vi "Insight OCT.vi"() -> ()   [LabVIEW 2014]
doc: "I. Description:\nThis example demonstrates how to acquire a continuous amount of data (Waveform) using the DAQ device's internal clock.\n\nII. Instructions for Running:\n1. Create an analog input voltage channel.\n2. Set the rate for the sample clock. Additionally, define the sample mode to be continuous.\n3. Call the Start VI to start the acquisition.\n4. Read the waveform data in a loop until the user hits the stop button or an error occurs.\nNote: This example reads data from one or more channels and returns an array of data. Use the Index Array function to access an individual channel of data.\n5. Call the Clear Task VI to clear the Task.\n6. Use the popup dialog box to display an error if any.\n\nIV. I/O Connections Overview:\nMake sure your signal input terminal matches the Physical Channel I/O Control. For further connection information, refer to your hardware reference manual."
uses:
  Type Defs/OCT Hardware States.ctl
  Classes/DAQ/DAQ Control Functional Global States.ctl
  Classes/Processing/Intensity/Intensity Processing.lvclass
  Classes/Galvo/NI Galvo/NI Galvo.lvclass
  Classes/DAQ/DAQ Class.lvclass
  Classes/DAQ/ATS9350/ATS9350.lvclass
  Classes/Laser/Insite/Insight.lvclass
  Type Defs/OCT DAQ Channel Data Type.ctl
  Classes/Galvo/Scanning Cluster.ctl
  Classes/Galvo/Galvo.lvclass
  Classes/DAQ/Clock Control.ctl
  Classes/DAQ/Trigger Source.ctl
  Classes/DAQ/Trigger Slope.ctl
  Classes/DAQ/DAQ Parameters.ctl
panel:
  out "Initial DAQ Parameters":T1={"Points Per A-Scan"=1024, "A-Scans Per B-Scan"=250, "Number of B-Scans"=1, "A-Scans Per Transfer"=1, "Trigger Voltage"=0.0, "Trigger Source"=enum."External", "Trigger Slope"=enum."Rising", "Channel"=enum."Channel 1", "Clock"=enum."Internal Clock", "Bits per Sample"=0.0, "Range"=0.0}
  in  "Laser Status":string
  out "Single A-Scan":u16[](graph)
  in  "Scanning Parameters":T6={"Fast Axis Offset"=0.0, "Slow Axis Offset"=0.0, "Slow Axis Amp"=2.0, "Fast Axis Amp"=2.0, "Scan Pattern"=enum."Raster"} {"Fast Axis Amp" max=20 format="%#.2f"; "Slow Axis Amp" max=20 format="%#.2f"; "Slow Axis Offset" max=10 format="%#.2f"; "Fast Axis Offset" max=10 format="%#.2f"}
  out "Log10?":bool
  in  "OCT Hardware States":T7
  out "Background Array":u16[](array[numeric])
  in  "Save Sweep Button":bool
  in  "Data Format":T4
  in  "Save Sweep":bool
  in  "Stop Button":bool
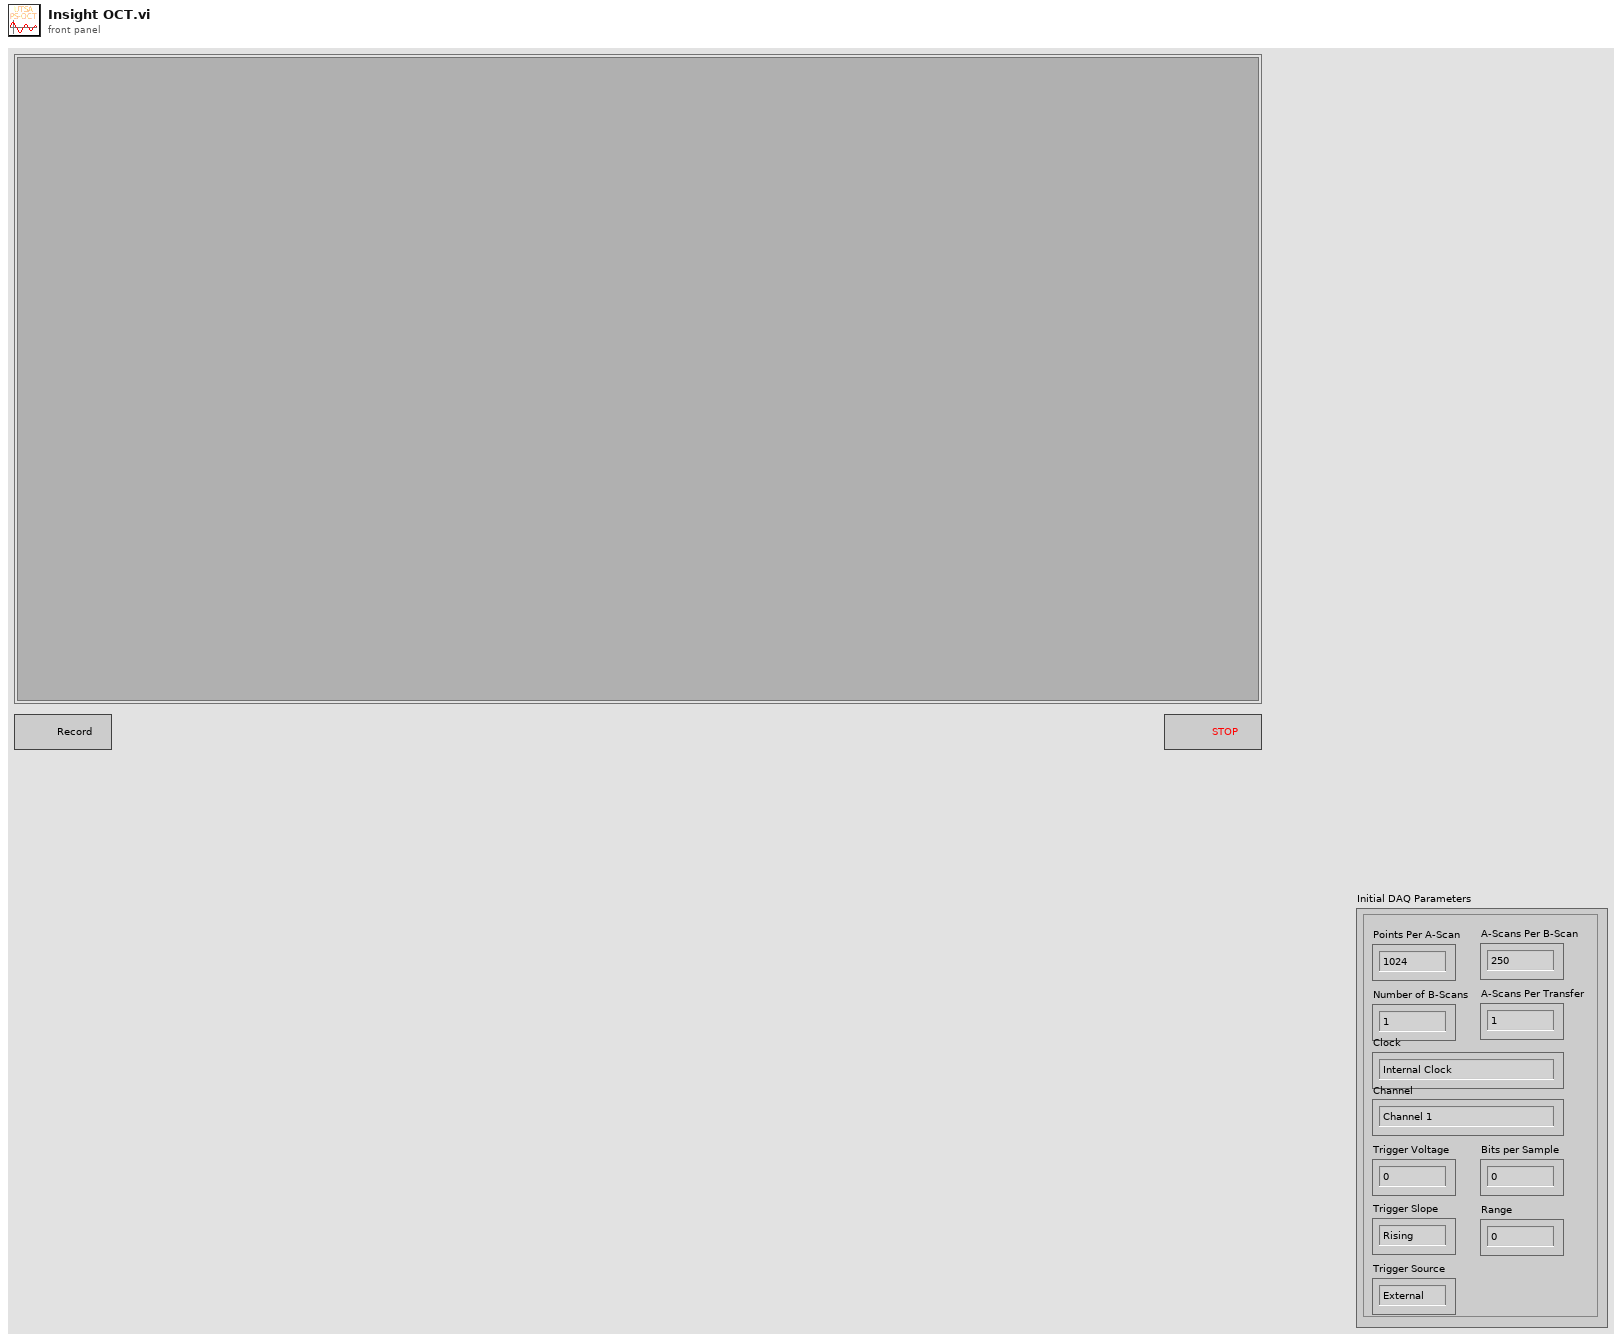
[diagram p1: front panel]
types:
  T1 = typedef "DAQ Class.lvclass/DAQ Parameters.ctl" = cluster{"Points Per A-Scan":u32, "A-Scans Per B-Scan":u32, "Number of B-Scans":u32, "A-Scans Per Transfer":u32, "Trigger Voltage":sgl, "Trigger Source":T2, "Trigger Slope":T3, "Channel":T4, "Clock":T5, "Bits per Sample":dbl, "Range":dbl}
  T2 = typedef "DAQ Class.lvclass/Trigger Source.ctl" = enum16{"External", "Channel A", "Channel B"}
  T3 = typedef "DAQ Class.lvclass/Trigger Slope.ctl" = enum16{"Rising", "Falling"}
  T4 = typedef "OCT DAQ Channel Data Type.ctl" = enum16{"Channel 1", "Channel 2", "Channel 1 and 2"}
  T5 = typedef "DAQ Class.lvclass/Clock Control.ctl" = enum16{"Internal Clock", "External Clock"}
  T6 = typedef "Galvo.lvclass/Scanning Cluster.ctl" = cluster{"Fast Axis Offset":sgl, "Slow Axis Offset":sgl, "Slow Axis Amp":sgl, "Fast Axis Amp":sgl, "Scan Pattern":enum16{"Raster"}}
  T7 = typedef "OCT Hardware States.ctl" = enum16{"Acquire Data", "Initialize Laser", "Initialize Galvos", "Startup", "Reset DAQ", "Background Subtraction", "Acquire Background", "Update DAQ Parameters", "Stop", "Set Clock", "Initialize DAQ", "Set Resampling Array", "Save Sweep", "Configure Laser", "128 x 128", "512 x 1", "512 x 512", "Review Data", "Configure Trigger", "Update Galvos"}
  T8 = typedef "DAQ Control Functional Global States.ctl" = enum16{"Status", "Set Processing Finished", "Reset", "Clear", "Set DAQ Finished"}
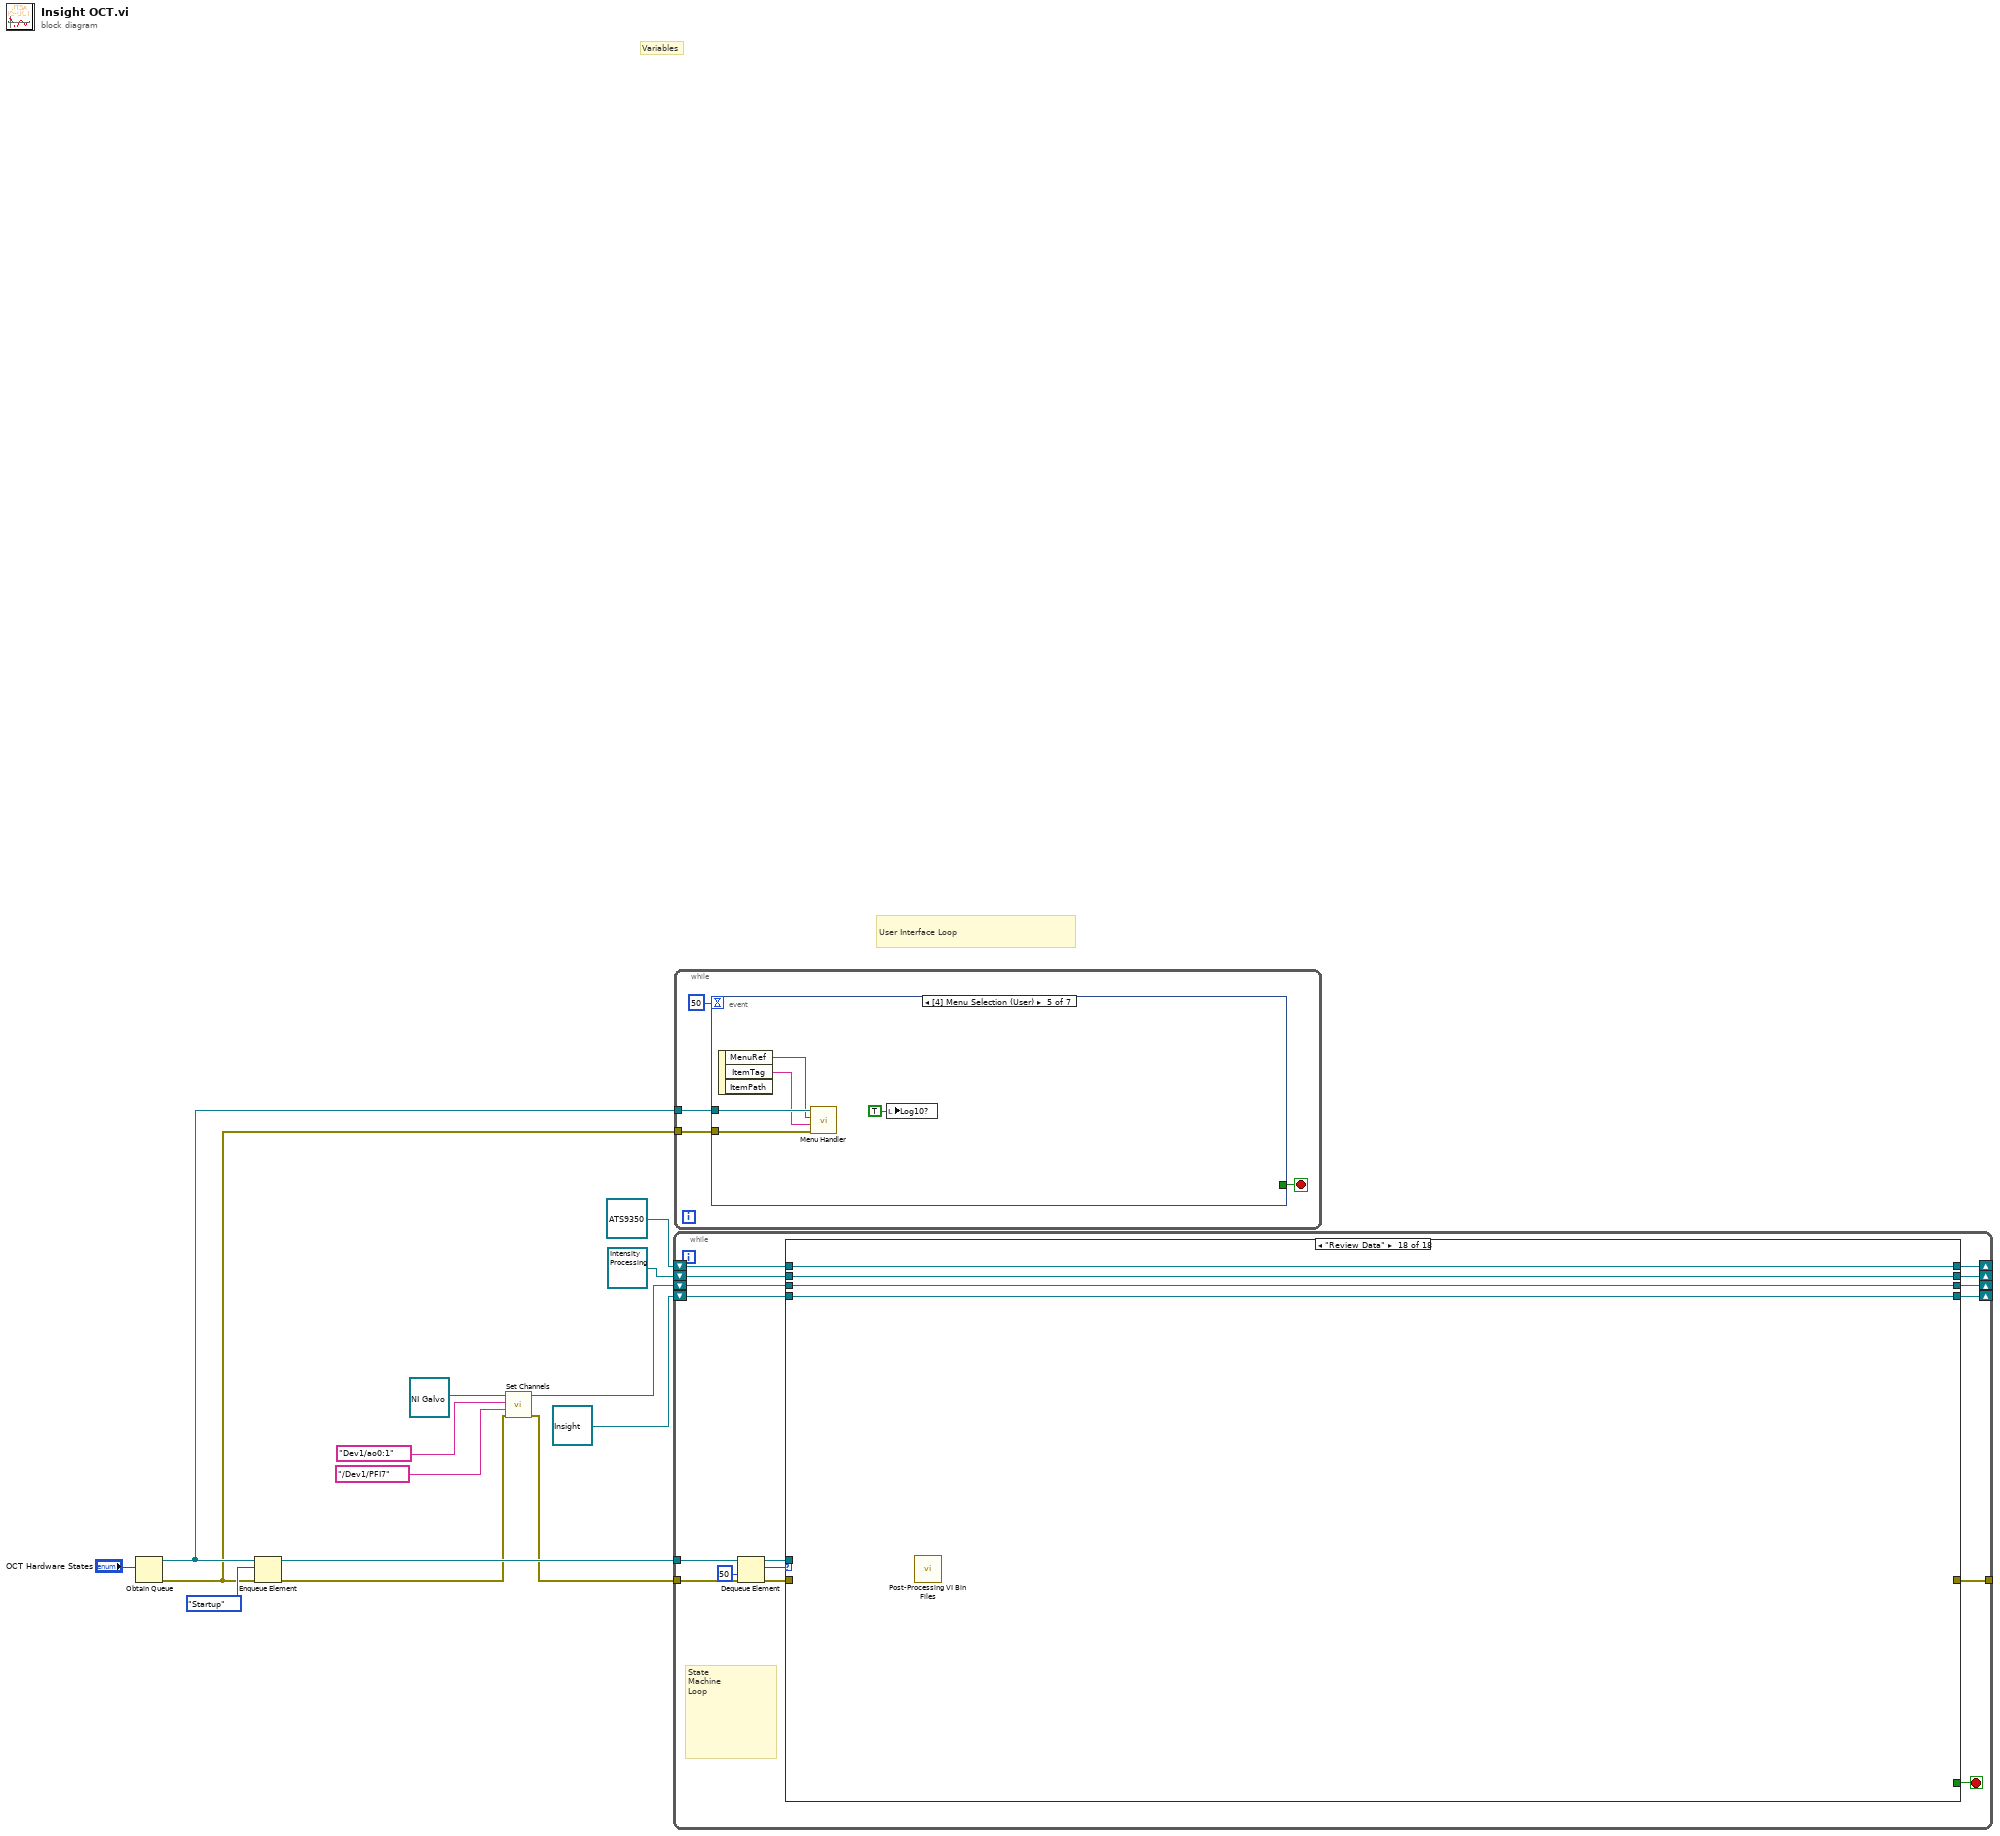
[diagram p0: block diagram]
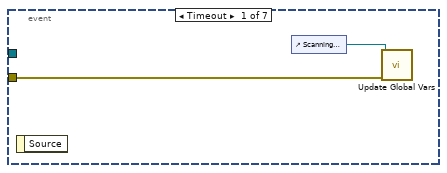
[diagram p2: hidden frame]
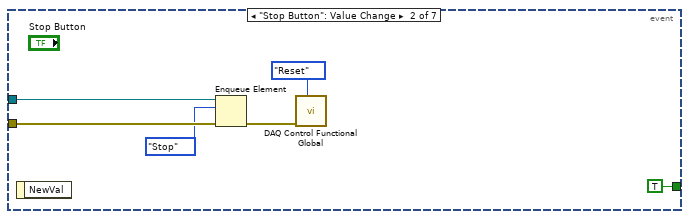
[diagram p3: hidden frame]
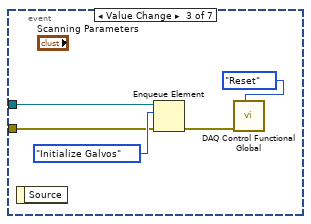
[diagram p4: hidden frame]
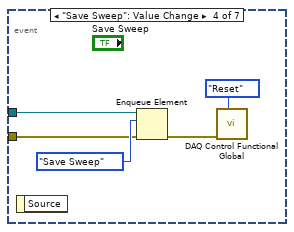
[diagram p5: hidden frame]
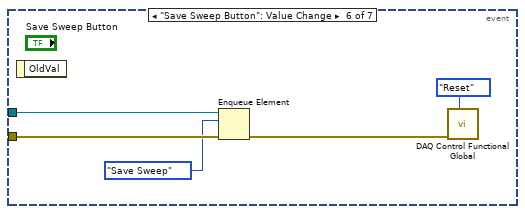
[diagram p6: hidden frame]
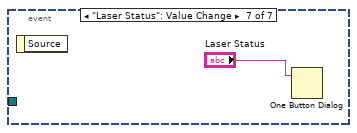
[diagram p7: hidden frame]
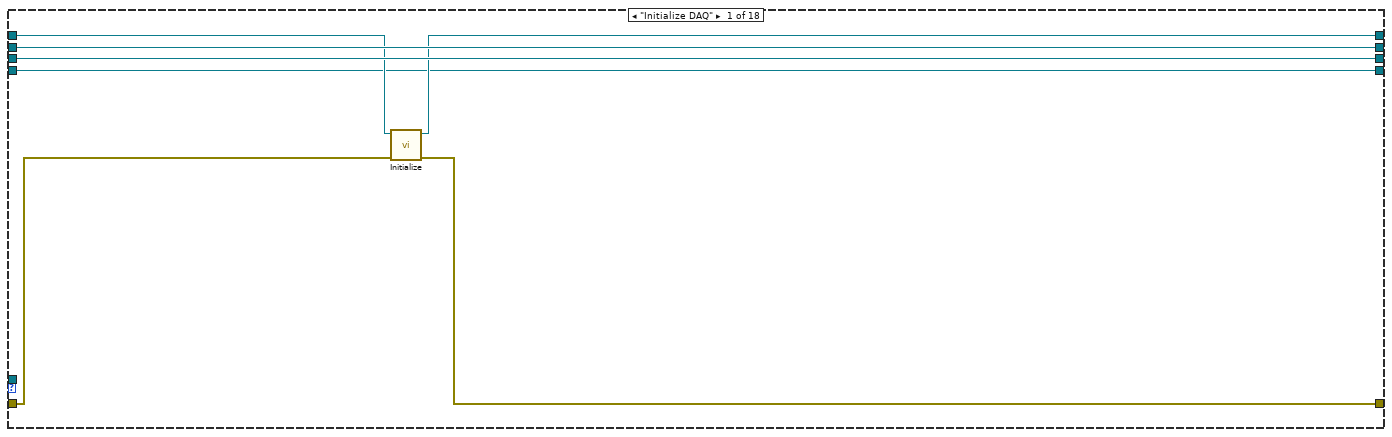
[diagram p8: hidden frame]
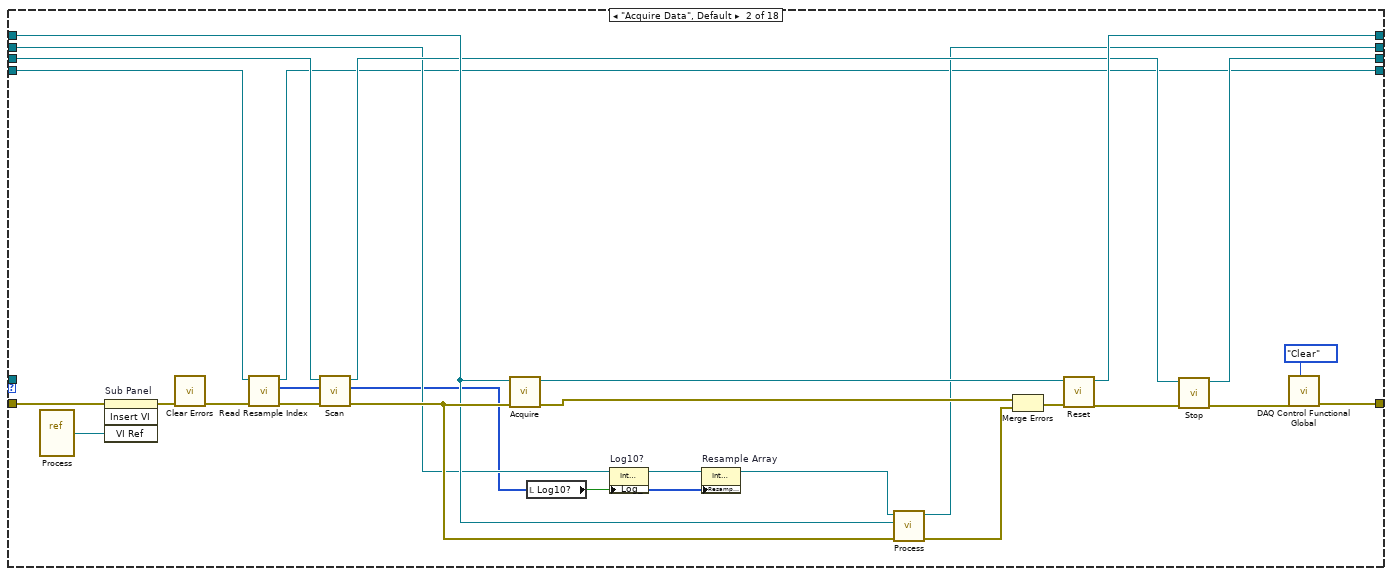
[diagram p9: hidden frame]
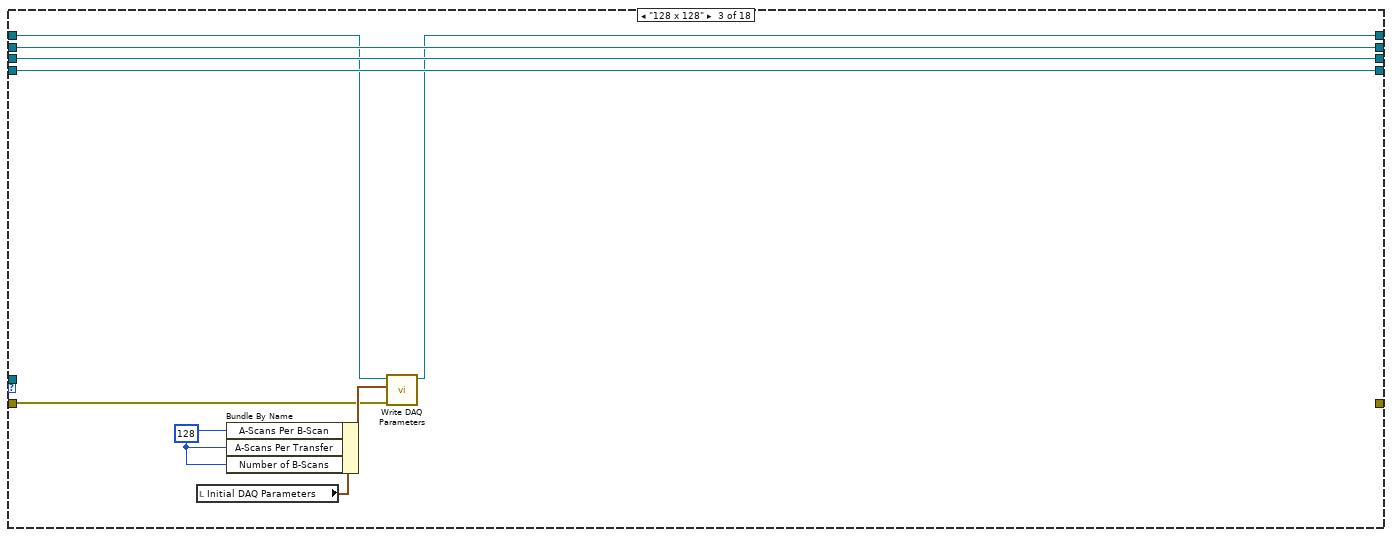
[diagram p10: hidden frame]
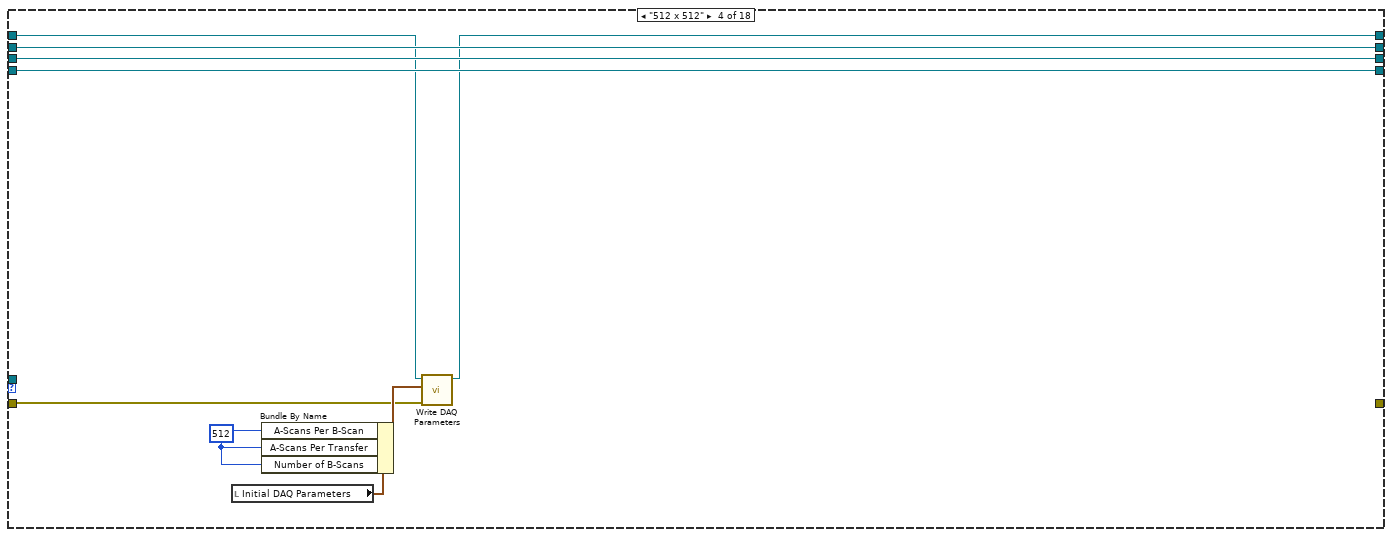
[diagram p11: hidden frame]
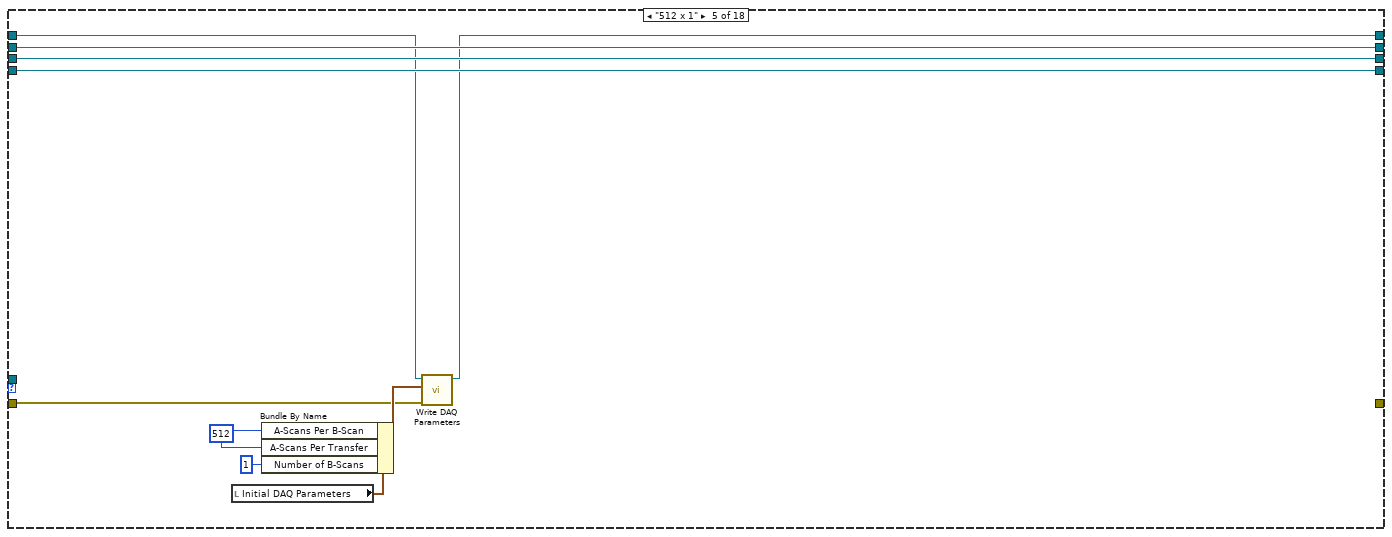
[diagram p12: hidden frame]
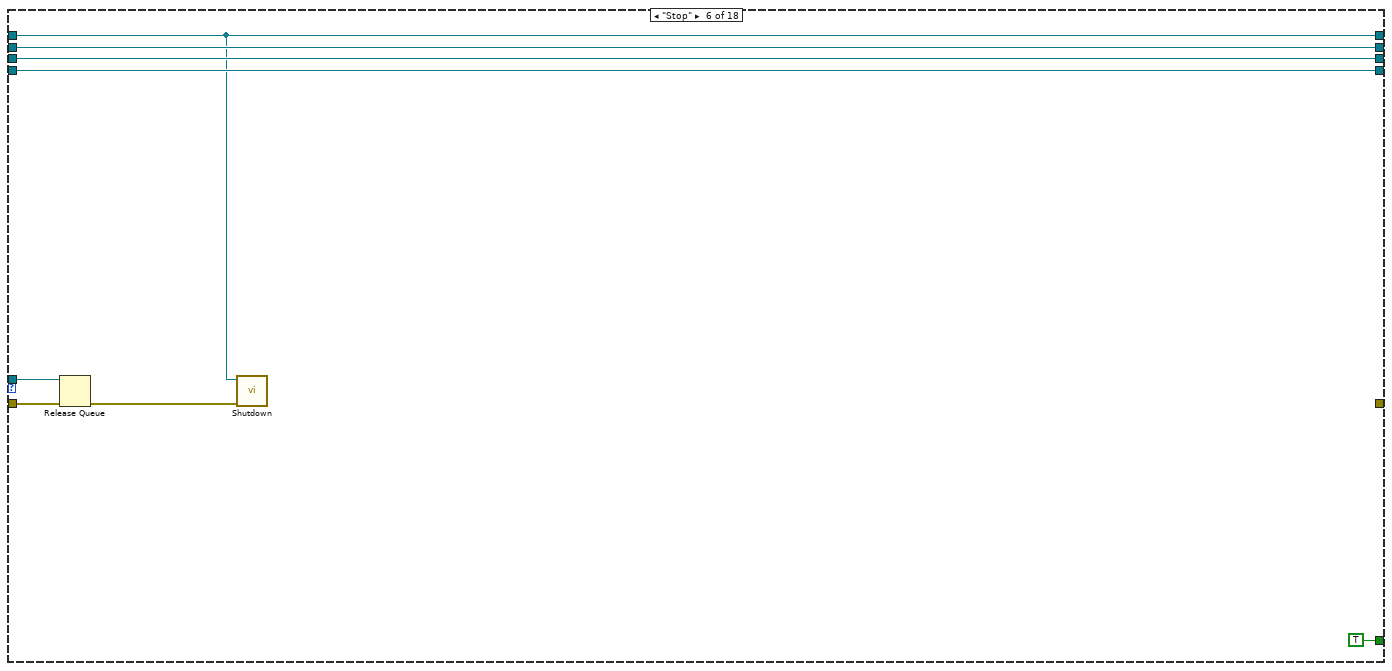
[diagram p13: hidden frame]
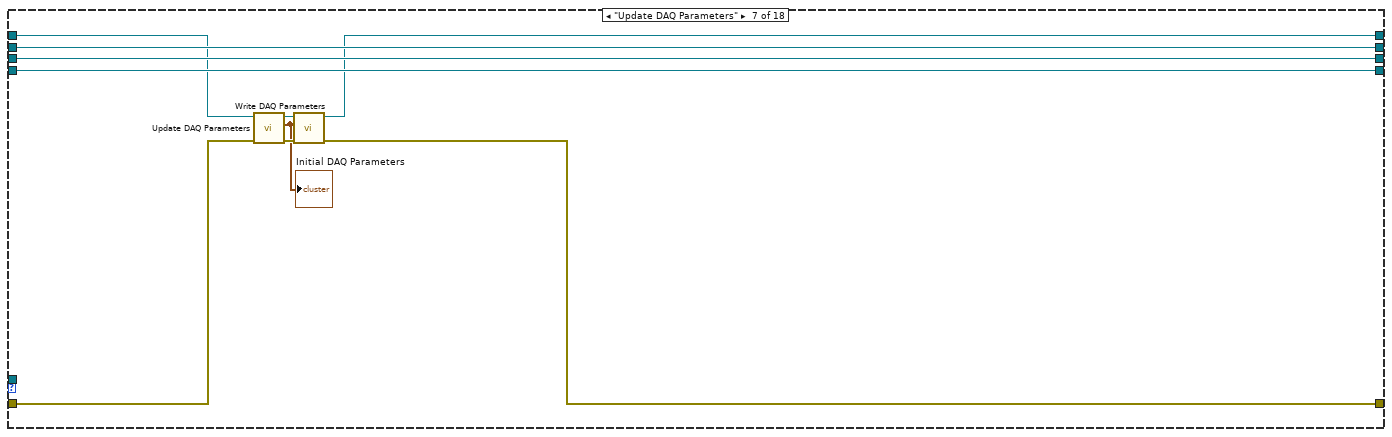
[diagram p14: hidden frame]
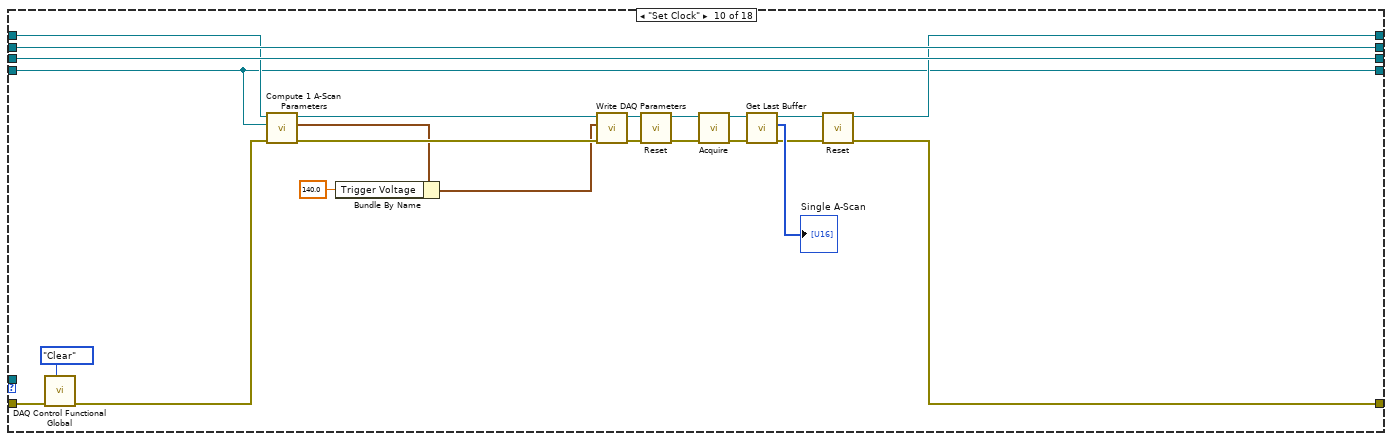
[diagram p17: hidden frame]
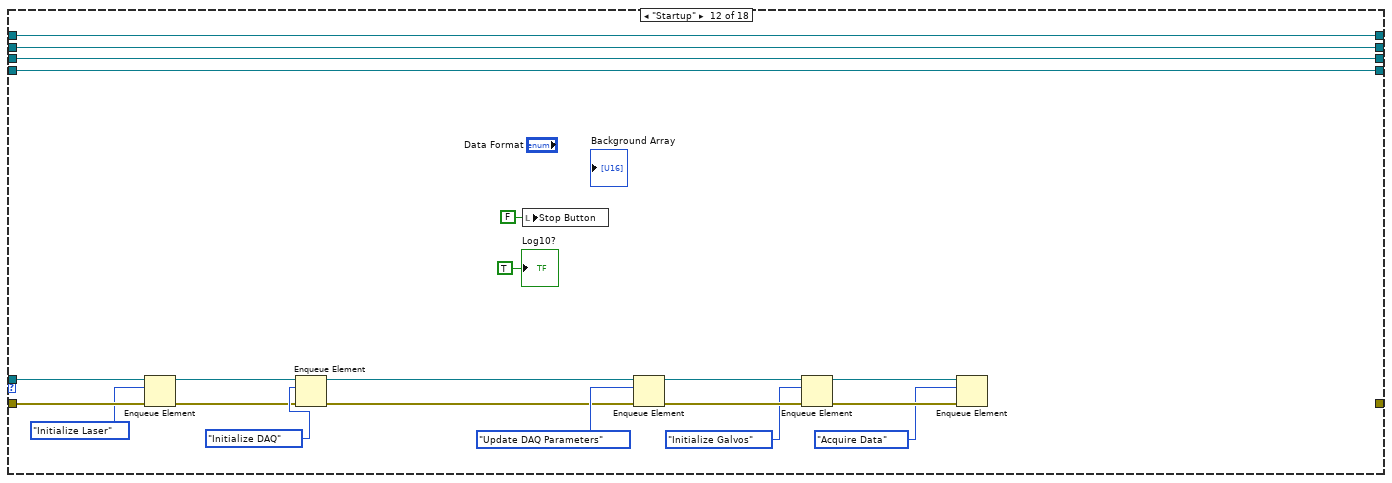
[diagram p19: hidden frame]
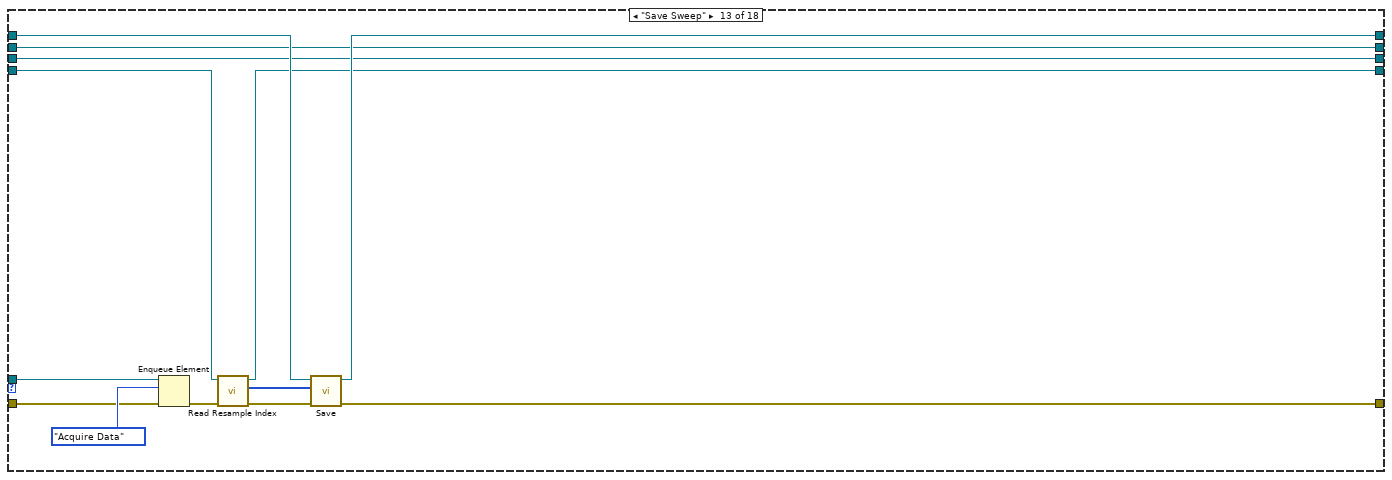
[diagram p20: hidden frame]
diagram:
  # "User Interface Loop"
  # "Variables"
  n1 = Obtain Queue(element data type="OCT Hardware States") -> (queue out=w12:refnum<queue>, error out=w10:errorcluster)  [unwired: 4 in, 1 out]
  n2 = Enqueue Element(queue=w12, element=OCT_Hardware_States."Startup", error in (no error)=w10) -> (queue out=w13:refnum<queue>, error out=w7:errorcluster)  [unwired: 1 in, 1 out]
  n3 = call-dynamic "Set Channels.vi"("error in (no error)"=w7, "Trigger Source"=tag "/Dev1/PFI7", "Analog Output"=tag "Dev1/ao0:1", "NI Galvo in"=refnum<class "NI Galvo.lvclass"> refnum ("NI Galvo.lvclass")) -> ("error out"=w6:errorcluster, "NI Galvo out"=w5:refnum<class "NI Galvo.lvclass">)  [unwired: 6 in]
  n4 = while {
    tunnel: w13 -> [w30]
    tunnel: w6 -> [w25]
    tunnel: [w26] -> _
    shift-right: [w22] -> _
    shift-left: refnum<class "ATS9350.lvclass"> refnum ("ATS9350.lvclass") -> [w23]
    shift-right: [w18] -> _
    shift-left: refnum<class "Intensity Processing.lvclass"> refnum ("Intensity Processing.lvclass") -> [w21]
    shift-right: [w17] -> _
    shift-left: w5 -> [w20]
    shift-right: [w16] -> _
    shift-left: refnum<class "Insight.lvclass"> refnum ("Insight.lvclass") -> [w19]
    stop <- w15 stop-if-true
    # "State\nMachine\nLoop"
    n5 = Dequeue Element(queue=w30, timeout in ms (-1)=50, error in (no error)=w25) -> (queue out=w28:refnum<queue>, element=w24:T7, error out=w29:errorcluster)  [unwired: 1 out]
    n6 = case shown="\"Review Data\"" w24 {
      tunnel: w29 -> [w32 w54 w67 w76 w86 w99 w110 _ _ w138 _ w151 w178 w186 _ w200 w210 _]
      tunnel: w28 -> [_ _ _ _ _ w100 _ _ _ _ _ w152 w177 _ _ _ _ _]
      tunnel: [w37 w63 _ _ _ _ w102 _ _ w120 _ _ w176 w189 _ w198 w205 _] -> w26
      tunnel: w23 -> [w34 w51 w66 w75 w85 w94 w104 w114 w118 w128 w145 w156 w175 w181 w196 w203 w213 w217]
      tunnel: [w33 w50 w65 w74 w84 w94 w103 w114 w118 w121 w145 w156 w174 w180 w196 w203 w213 w217] -> w22
      tunnel: w21 -> [w36 w47 w73 w82 w92 w97 w107 w113 w117 w130 w144 w155 w173 w185 w195 w202 w212 w216]
      tunnel: w20 -> [w35 w52 w72 w81 w91 w96 w106 w112 w116 w129 w143 w154 w172 w183 w194 w201 w211 w215]
      tunnel: w19 -> [w31 w42 w71 w80 w90 w95 w105 w111 w115 w119 w142 w153 w169 w184 w193 w199 w207 w214]
      tunnel: [w36 w46 w73 w82 w92 w97 w107 w113 w117 w130 w144 w155 w173 w185 w195 w202 w212 w216] -> w18
      tunnel: [w35 w48 w72 w81 w91 w96 w106 w112 w116 w129 w143 w154 w172 w182 w194 w201 w211 w215] -> w17
      tunnel: [w31 w41 w71 w80 w90 w95 w105 w111 w115 w119 w142 w153 w168 w184 w193 w197 w206 w214] -> w16
      tunnel: [_ _ _ _ _ TRUE _ _ _ _ _ _ _ _ _ _ _ _] -> w15
      frame "Initialize DAQ" {
        n7 = call-dynamic "Initialize.vi"("error in (no error)"=w32, "ATS9350 in"=w34) -> ("error out"=w37:errorcluster, "ATS9350 out"=w33:refnum<class "ATS9350.lvclass">)  [unwired: 8 in]
      }
      frame "Acquire Data", Default {
        n8 = vi-ref "Process.vi"() -> (w53:refnum<vi>)
        n9 = invoke on="Sub Panel" class="SubPanel" method="Insert VI"(error in=w54, "VI Ref"=w53) -> (error out=w45:errorcluster)  [unwired: 2 in, 3 out]
        n10 = call <vilib>:"Clear Errors.vi"("error in (no error)"=w45) -> ("error out"=w44:errorcluster)  [unwired: 5 in, 1 out]
        n11 = call-dynamic "Read Resample Index.vi"("error in (no error)"=w44, "Laser in"=w42) -> ("error out"=w43:errorcluster, "Resample Index"=w39:u32[], "Laser out"=w41:refnum<class "Insight.lvclass">)  [unwired: 7 in]
        n12 = call-dynamic "Scan.vi"("error in (no error)"=w43, "NI Galvo in"=w52) -> ("error out"=w57:errorcluster, "NI Galvo out"=w49:refnum<class "NI Galvo.lvclass">)  [unwired: 8 in]
        n13 = call-dynamic "Acquire.vi"("error in (no error)"=w57, "ATS9350 in"=w51) -> ("error out"=w61:errorcluster, "ATS9350 out"=w59:refnum<class "ATS9350.lvclass">)  [unwired: 8 in]
        n14 = local read "Log10?"() -> (w58:bool)
        n15 = property on="Log10?" class="Intensity Processing.lvclass"(reference=w47, "Log_"=w58) -> (reference out=w40:refnum<class "Intensity Processing.lvclass">)  [unwired: 1 in, 1 out]
        n16 = property on="Resample Array" class="Intensity Processing.lvclass"(reference=w40, "Resample Array"=w39) -> (reference out=w38:refnum<class "Intensity Processing.lvclass">)  [unwired: 1 in, 1 out]
        n17 = call-dynamic "Process.vi"("error in (no error)"=w57, "DAQ Class.lvclass"=w51, "Intensity Processing in"=w38) -> ("error out"=w62:errorcluster, "Intensity Processing out"=w46:refnum<class "Intensity Processing.lvclass">)  [unwired: 7 in]
        n18 = Merge Errors(w61, w62) -> (w60:errorcluster)
        n19 = call-dynamic "Reset.vi"("error in (no error)"=w60, "ATS9350 in"=w59) -> ("error out"=w56:errorcluster, "ATS9350 out"=w50:refnum<class "ATS9350.lvclass">)  [unwired: 8 in]
        n20 = call-dynamic "Stop.vi"("error in (no error)"=w56, "NI Galvo in"=w49) -> ("error out"=w55:errorcluster, "NI Galvo out"=w48:refnum<class "NI Galvo.lvclass">)  [unwired: 8 in]
        n21 = call "DAQ Control Functional Global.vi"("State"=DAQ_Control_Functional_Global_States."Clear", "Error In"=w55) -> ("Error Out"=w63:errorcluster)  [unwired: 6 in, 3 out]
      }
      frame "128 x 128" {
        w69 = u32 128 ("A-Scans Per B-Scan")
        n22 = local read "Initial DAQ Parameters"() -> (w70:T1)
        n23 = Bundle By Name(cluster=w70, "A-Scans Per B-Scan"=w69, "A-Scans Per Transfer"=w69, "Number of B-Scans"=w69) -> (w68:T1)
        n24 = call-dynamic "Write DAQ Parameters.vi"("error in (no error)"=w67, "DAQ Parameters"=w68, "ATS9350 in"=w66) -> ("ATS9350 out"=w65:refnum<class "ATS9350.lvclass">)  [unwired: 7 in, 1 out]
      }
      frame "512 x 512" {
        w78 = u32 512 ("A-Scans Per B-Scan")
        n25 = local read "Initial DAQ Parameters"() -> (w79:T1)
        n26 = Bundle By Name(cluster=w79, "A-Scans Per B-Scan"=w78, "A-Scans Per Transfer"=w78, "Number of B-Scans"=w78) -> (w77:T1)
        n27 = call-dynamic "Write DAQ Parameters.vi"("error in (no error)"=w76, "DAQ Parameters"=w77, "ATS9350 in"=w75) -> ("ATS9350 out"=w74:refnum<class "ATS9350.lvclass">)  [unwired: 7 in, 1 out]
      }
      frame "512 x 1" {
        w88 = u32 512 ("A-Scans Per B-Scan")
        n28 = local read "Initial DAQ Parameters"() -> (w89:T1)
        n29 = Bundle By Name(cluster=w89, "A-Scans Per B-Scan"=w88, "A-Scans Per Transfer"=w88, "Number of B-Scans"=u32 1) -> (w87:T1)
        n30 = call-dynamic "Write DAQ Parameters.vi"("error in (no error)"=w86, "DAQ Parameters"=w87, "ATS9350 in"=w85) -> ("ATS9350 out"=w84:refnum<class "ATS9350.lvclass">)  [unwired: 7 in, 1 out]
      }
      frame "Stop" {
        n31 = Release Queue(queue=w100, error in (no error)=w99) -> (error out=w98:errorcluster)  [unwired: 1 in, 2 out]
        n32 = call-dynamic "Shutdown.vi"("error in (no error)"=w98, "ATS9350 in"=w94) -> ()  [unwired: 8 in, 2 out]
      }
      frame "Update DAQ Parameters" {
        n33 = call-dynamic "Update DAQ Parameters.vi"("error in (no error)"=w110, "DAQ Class in"=w104) -> ("error out"=w108:errorcluster, "DAQ Parameters Out"=w101:T1, "DAQ Class out"=w109:refnum<class "ATS9350.lvclass">)  [unwired: 7 in]
        "Initial DAQ Parameters" <- w101
        n34 = call-dynamic "Write DAQ Parameters.vi"("error in (no error)"=w108, "DAQ Parameters"=w101, "ATS9350 in"=w109) -> ("error out"=w102:errorcluster, "ATS9350 out"=w103:refnum<class "ATS9350.lvclass">)  [unwired: 7 in]
      }
      frame "Background Subtraction" {
      }
      frame "Acquire Background" {
      }
      frame "Set Clock" {
        n35 = call "DAQ Control Functional Global.vi"("State"=DAQ_Control_Functional_Global_States."Clear", "Error In"=w138) -> ("Error Out"=w137:errorcluster)  [unwired: 6 in, 3 out]
        n36 = call "Compute 1 A-Scan Parameters.vi"("error in (no error)"=w137, "Laser In"=w119, "DAQ Class.lvclass"=w128) -> ("error out"=w131:errorcluster, "DAQ Parameters"=w127:T1, "DAQ Class.lvclass 2"=w132:refnum<class "ATS9350.lvclass">)  [unwired: 6 in]
        n37 = Bundle By Name(cluster=w127, "Trigger Voltage"=sgl 140.0) -> (w125:T1)
        n38 = call-dynamic "Write DAQ Parameters.vi"("error in (no error)"=w131, "DAQ Parameters"=w125, "ATS9350 in"=w132) -> ("error out"=w136:errorcluster, "ATS9350 out"=w135:refnum<class "ATS9350.lvclass">)  [unwired: 7 in]
        n39 = call-dynamic "Reset.vi"("error in (no error)"=w136, "ATS9350 in"=w135) -> ("error out"=w133:errorcluster, "ATS9350 out"=w134:refnum<class "ATS9350.lvclass">)  [unwired: 8 in]
        n40 = call-dynamic "Acquire.vi"("error in (no error)"=w133, "ATS9350 in"=w134) -> ("error out"=w140:errorcluster, "ATS9350 out"=w141:refnum<class "ATS9350.lvclass">)  [unwired: 8 in]
        n41 = call-dynamic "Get Last Buffer.vi"("error in (no error)"=w140, "DAQ Class in"=w141) -> ("error out"=w123:errorcluster, "Last Buffer"=→"Single A-Scan":u16[], "DAQ Class out"=w122:refnum<class "ATS9350.lvclass">)  [unwired: 7 in]
        n42 = call-dynamic "Reset.vi"("error in (no error)"=w123, "ATS9350 in"=w122) -> ("error out"=w120:errorcluster, "ATS9350 out"=w121:refnum<class "ATS9350.lvclass">)  [unwired: 8 in]
      }
      frame "Set Resampling Array" {
      }
      frame "Startup" {
        n43 = Enqueue Element(queue=w152, element=OCT_Hardware_States."Initialize Laser", error in (no error)=w151) -> (queue out=w149:refnum<queue>, error out=w150:errorcluster)  [unwired: 1 in, 1 out]
        n44 = Enqueue Element(queue=w149, element=OCT_Hardware_States."Initialize DAQ", error in (no error)=w150) -> (queue out=w147:refnum<queue>, error out=w146:errorcluster)  [unwired: 1 in, 1 out]
        n45 = local write "Stop Button"(FALSE ("Sweep Ready for saving")) -> ()
        n46 = Enqueue Element(queue=w147, element=OCT_Hardware_States."Update DAQ Parameters", error in (no error)=w146) -> (queue out=w164:refnum<queue>, error out=w163:errorcluster)  [unwired: 1 in, 1 out]
        n47 = Enqueue Element(queue=w164, element=OCT_Hardware_States."Initialize Galvos", error in (no error)=w163) -> (queue out=w159:refnum<queue>, error out=w158:errorcluster)  [unwired: 1 in, 1 out]
        n48 = Enqueue Element(queue=w159, element=OCT_Hardware_States."Acquire Data", error in (no error)=w158) -> ()  [unwired: 1 in, 3 out]
        "Log10?" <- TRUE ("Log10?")
      }
      frame "Save Sweep" {
        n49 = Enqueue Element(queue=w177, element=OCT_Hardware_States."Acquire Data", error in (no error)=w178) -> (error out=w171:errorcluster)  [unwired: 1 in, 2 out]
        n50 = call-dynamic "Read Resample Index.vi"("error in (no error)"=w171, "Laser in"=w169) -> ("error out"=w170:errorcluster, "Resample Index"=w167:u32[], "Laser out"=w168:refnum<class "Insight.lvclass">)  [unwired: 7 in]
        n51 = call-dynamic "Save.vi"("error in (no error)"=w170, "Resampling Array"=w167, "DAQ Class in"=w175) -> ("error out"=w176:errorcluster, "DAQ Class out"=w174:refnum<class "ATS9350.lvclass">)  [unwired: 7 in]
      }
      frame "Initialize Galvos" {
        n52 = call-dynamic "Read DAQ Parameters.vi"("error in (no error)"=w186, "ATS9350 in"=w181) -> ("error out"=w187:errorcluster, "DAQ Parameters"=w188:T1, "ATS9350 out"=w180:refnum<class "ATS9350.lvclass">)  [unwired: 7 in]
        n53 = local read "Scanning Parameters"() -> (w192:T6)
        n54 = call-dynamic "Configure.vi"("error in (no error)"=w187, "DAQ Parameters"=w188, "Scanning Parameters"=w192, "NI Galvo in"=w183) -> ("error out"=w191:errorcluster, "NI Galvo out"=w190:refnum<class "NI Galvo.lvclass">)  [unwired: 6 in]
        n55 = call-dynamic "Initialize.vi"("error in (no error)"=w191, "NI Galvo in"=w190) -> ("error out"=w189:errorcluster, "NI Galvo out"=w182:refnum<class "NI Galvo.lvclass">)  [unwired: 8 in]
      }
      frame "Reset DAQ" {
      }
      frame "Configure Laser" {
        n56 = call-dynamic "Configure.vi"("error in (no error)"=w200, "Insight in"=w199) -> ("error out"=w198:errorcluster, "Insight out"=w197:refnum<class "Insight.lvclass">)  [unwired: 8 in]
      }
      frame "Initialize Laser" {
        n57 = call-dynamic "Init.vi"("error in (no error)"=w210, "Insite in"=w207) -> ("error out"=w208:errorcluster, "Insite out"=w209:refnum<class "Insight.lvclass">)  [unwired: 8 in]
        n58 = call-dynamic "Read Status.vi"("error in (no error)"=w208, "Laser in"=w209) -> ("error out"=w205:errorcluster, "Status"=w204:string, "Laser out"=w206:refnum<class "Insight.lvclass">)  [unwired: 7 in]
        n59 = local write "Laser Status"(w204) -> ()
      }
      frame "Review Data" {
        n60 = call "Post-Processing VI Bin Files.vi"() -> ()  [unwired: 12 in]
      }
    }
  }
  n61 = while {
    tunnel: w12 -> [w221]
    tunnel: w10 -> [w220]
    stop <- w218 stop-if-true
    n62 = event shown="[4] Menu Selection (User)" {
      selector: _ -> [_ _ _ _ _ _ _]
      dyn-events: _ -> [_ _ _ _ _ _ _]
      timeout: 50 -> [_ _ _ _ _ _ _]
      tunnel: w221 -> [_ w228 w231 w236 w244 w246 _]
      tunnel: w220 -> [w222 w229 w232 w237 w243 w248 _]
      tunnel: [_ TRUE _ _ _ _ _] -> w218
      event Timeout {
        n63 = event-data() -> ()  [unwired: 1 in, 1 out]
        n64 = control-ref of="Scanning Parameters"() -> (w223:refnum<vi>)
        n65 = call "Update Global Vars.vi"("Error In"=w222, "Cluster in"=w223) -> ()  [unwired: 9 in, 1 out]
      }
      event "Stop Button": Value Change {
        n66 = event-data() -> ()  [unwired: 1 in, 1 out]
        n67 = Enqueue Element(queue=w228, element=OCT_Hardware_States."Stop", error in (no error)=w229) -> (error out=w226:errorcluster)  [unwired: 1 in, 2 out]
        n68 = call "DAQ Control Functional Global.vi"("State"=DAQ_Control_Functional_Global_States."Reset", "Error In"=w226) -> ()  [unwired: 6 in, 4 out]
      }
      event Value Change {
        n69 = event-data() -> ()  [unwired: 1 in, 1 out]
        n70 = Enqueue Element(queue=w231, element=OCT_Hardware_States."Initialize Galvos", error in (no error)=w232) -> (error out=w233:errorcluster)  [unwired: 1 in, 2 out]
        n71 = call "DAQ Control Functional Global.vi"("State"=DAQ_Control_Functional_Global_States."Reset", "Error In"=w233) -> ()  [unwired: 6 in, 4 out]
      }
      event "Save Sweep": Value Change {
        n72 = event-data() -> ()  [unwired: 1 in, 1 out]
        n73 = Enqueue Element(queue=w236, element=OCT_Hardware_States."Save Sweep", error in (no error)=w237) -> (error out=w235:errorcluster)  [unwired: 1 in, 2 out]
        n74 = call "DAQ Control Functional Global.vi"("State"=DAQ_Control_Functional_Global_States."Reset", "Error In"=w235) -> ()  [unwired: 6 in, 4 out]
      }
      event Menu Selection (User) {
        n75 = event-data() -> ("MenuRef"=w241:refnum<k9>, "ItemTag"=w242:string)  [unwired: 1 in, 1 out]
        n76 = call "Menu Handler.vi"("error in (no error)"=w243, "ItemTag"=w242, "Menu in"=w241, "queue in"=w244) -> ()  [unwired: 6 in, 2 out]
        n77 = local write "Log10?"(TRUE ("Log10?")) -> ()
      }
      event "Save Sweep Button": Value Change {
        n78 = event-data() -> ()  [unwired: 1 in, 1 out]
        n79 = Enqueue Element(queue=w246, element=OCT_Hardware_States."Save Sweep", error in (no error)=w248) -> (error out=w247:errorcluster)  [unwired: 1 in, 2 out]
        n80 = call "DAQ Control Functional Global.vi"("State"=DAQ_Control_Functional_Global_States."Reset", "Error In"=w247) -> ()  [unwired: 6 in, 4 out]
      }
      event "Laser Status": Value Change {
        n81 = event-data() -> ()  [unwired: 1 in, 1 out]
        n82 = One Button Dialog(message="Laser Status") -> ()  [unwired: 1 in, 1 out]
      }
    }
  }
